vi "Helper SubVI - Online Plot Buffered Peak Strip.vi"(5 "initialize? (F)":bool, 6 "block size":i32, 8 "error in (no error)":errorcluster, 11 "peak plot":cluster{"Ramp Pattern":dbl[], "X":dbl[]}[](array[cluster])) -> (0 "error out":errorcluster, 3 "plot data":cluster{"Ramp Pattern":dbl[], "trend":dbl[]}[](array[cluster]))   [LabVIEW 2023]
doc: "Generates online peak plots."
panel:
  in  "trend? (F)":bool
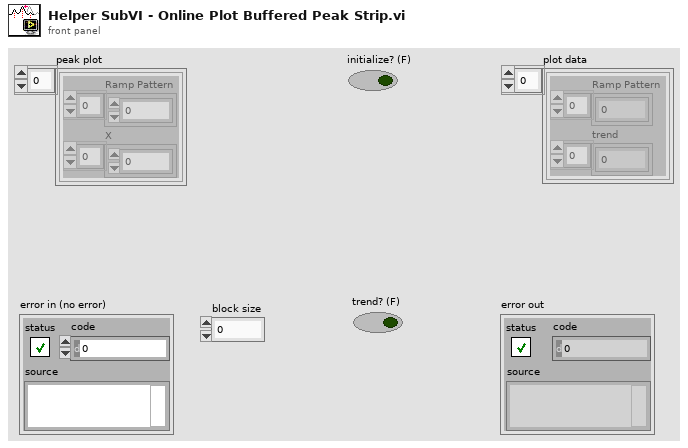
[diagram p1: front panel]
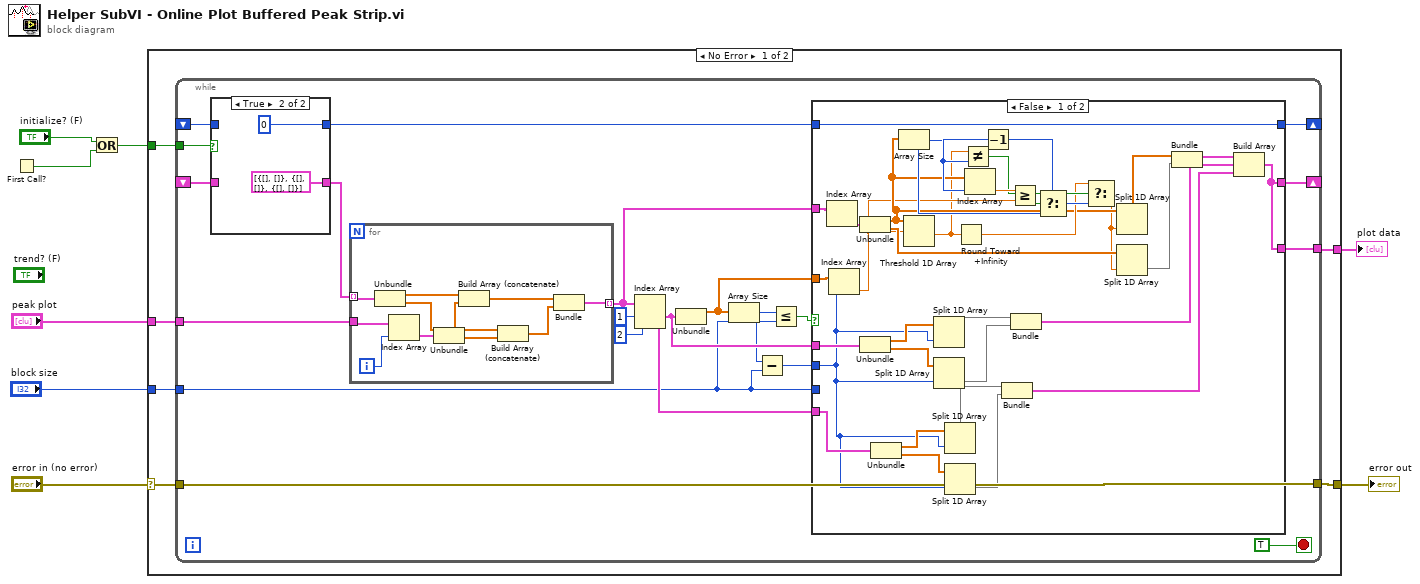
[diagram p0: block diagram]
diagram:
  n1 = First Call?() -> (First Call?: T/F=w7:bool)
  n2 = Or(x="initialize? (F)", y=w7) -> (x .or. y?=w5:bool)
  n3 = case shown="No Error" "error in (no error)" {
    selector: "error in (no error)" -> [w10 w86]
    tunnel: w5 -> [w14 _]
    tunnel: "peak plot" -> [w13 _]
    tunnel: "block size" -> [w12 _]
    tunnel: [w11 _] -> w2
    tunnel: [w9 w86] -> w1
    frame No Error {
      n4 = while {
        tunnel: w14 -> [w35]
        shift-right: [w24] -> _
        shift-left: _ -> [w33]
        shift-right: [w26] -> _
        shift-left: _ -> [w34]
        tunnel: w13 -> [w32]
        tunnel: w12 -> [w16]
        tunnel: [w28] -> w11
        tunnel: w10 -> [w18]
        tunnel: [w18] -> w9
        stop <- TRUE stop-if-true
        n5 = case shown="True" w35 {
          tunnel: [w82 cluster{"Ramp Pattern":dbl[], "X":dbl[]}[] [{"Ramp Pattern"=[], "X"=[]}, {"Ramp Pattern"=[], "X"=[]}, {"Ramp Pattern"=[], "X"=[]}] ("initialized array")] -> w25
          tunnel: [w83 0] -> w27
          tunnel: w34 -> [w83 _]
          tunnel: w33 -> [w82 _]
          frame False {
          }
          frame True {
          }
        }
        n6 = for {
          tunnel: w25 -> [w79] mode=indexing
          tunnel: w32 -> [w80]
          tunnel: [w71] -> w29 mode=indexing
          i -> [w81]
          n7 = Unbundle(w79) -> ("Ramp Pattern"=w77:dbl[], "X"=w74:dbl[])
          n8 = Index Array(array=w80, index=w81) -> (element=w78:cluster{"Ramp Pattern":dbl[], "X":dbl[]})
          n9 = Unbundle(w78) -> ("Ramp Pattern"=w76:dbl[], "X"=w75:dbl[])
          n10 = Build Array (concatenate)(w77, w76) -> (w73:dbl[])
          n11 = Build Array (concatenate)(w74, w75) -> (w72:dbl[])
          n12 = Bundle(w73, w72) -> (w71:cluster{dbl[], dbl[]})  [unwired: 1 in]
        }
        n13 = Index Array(array=w29, index #1=1 ("index"), index #2=2 ("index")) -> (element #1=w22:cluster{dbl[], dbl[]}, element #2=w20:cluster{dbl[], dbl[]})
        n14 = Unbundle(w22) -> (w23:dbl[])  [unwired: 1 out]
        n15 = Array Size(array=w23) -> (size(s)=w17:i32)
        n16 = Subtract(x=w17, y=w16) -> (x-y=w15:i32)
        n17 = Less Or Equal?(x=w17, y=w16) -> (x <= y?=w30:bool)
        n18 = case shown="False" w30 {
          tunnel: w29 -> [w67 w69]
          tunnel: [w48 w69] -> w28
          tunnel: w27 -> [w52 w70]
          tunnel: [w52 w70] -> w26
          tunnel: [w48 w69] -> w24
          tunnel: w23 -> [w68 _]
          tunnel: w16 -> [_ _]
          tunnel: w22 -> [w62 _]
          tunnel: w20 -> [w54 _]
          tunnel: w15 -> [w47 _]
          frame False {
            n19 = Index Array(array=w67) -> (element=w66:cluster{dbl[], dbl[]})  [unwired: 1 in]
            n20 = Index Array(array=w68, index=w47) -> (element=w38:dbl)
            n21 = Unbundle(w66) -> (w39:dbl[], w65:dbl[])
            n22 = Unbundle(w62) -> (w59:dbl[], w58:dbl[])
            n23 = Unbundle(w54) -> (w56:dbl[], w57:dbl[])
            n24 = Array Size(array=w39) -> (size(s)=w42:i32)
            n25 = Threshold 1D Array(2:w38, 3:w39) -> (0:w37:dbl)  [unwired: 1 in]
            n26 = Split 1D Array(array=w59, index=w47) -> (second subarray=w60:dbl[])  [unwired: 1 out]
            n27 = Split 1D Array(array=w58, index=w47) -> (second subarray=w61:dbl[])  [unwired: 1 out]
            n28 = Split 1D Array(array=w56, index=w47) -> (second subarray=w55:dbl[])  [unwired: 1 out]
            n29 = Split 1D Array(array=w57, index=w47) -> (second subarray=w53:dbl[])  [unwired: 1 out]
            n30 = Round Toward +Infinity(x=w37) -> (ceil(x): smallest int >= x=w40:dbl)
            n31 = Decrement(x=w42) -> (x-1=w43:i32)
            n32 = Not Equal?(x=w37, y=w43) -> (x != y?=w45:bool)
            n33 = Index Array(array=w39, index=w43) -> (element=w46:dbl)
            n34 = Bundle(w55, w53) -> (w49:cluster{dbl[], dbl[]})  [unwired: 1 in]
            n35 = Greater Or Equal?(x=w46, y=w38) -> (x >= y?=w44:bool)
            n36 = Bundle(w60, w61) -> (w50:cluster{dbl[], dbl[]})  [unwired: 1 in]
            n37 = Select(t=w43, s=w44, f=w42) -> (s? t:f=w41:i32)
            n38 = Select(t=w40, s=w45, f=w41) -> (s? t:f=w36:dbl)
            n39 = Split 1D Array(array=w39, index=w36) -> (second subarray=w64:dbl[])  [unwired: 1 out]
            n40 = Split 1D Array(array=w65, index=w36) -> (second subarray=w63:dbl[])  [unwired: 1 out]
            n41 = Bundle(w64, w63) -> (w51:cluster{dbl[], dbl[]})  [unwired: 1 in]
            n42 = Build Array(w51, w50, w49) -> (w48:cluster{dbl[], dbl[]}[])
          }
          frame True {
          }
        }
      }
    }
    frame Error {
    }
  }
  "plot data" <- w2
  "error out" <- w1
